vi "RT Driver VI.vi"(7 "Operation":T1, 11 "Device Reference in":T2 format="%.0x") -> (0 "Error Code":i32)   [LabVIEW 2021, in "Software Multi-Plex Engine.lvlib"]
uses:
  Software Multi-Plex Engine.lvlib
  <vilib>/NI VeriStand/Custom Device API/Custom Device Item Ref.ctl
  <vilib>/NI VeriStand/Custom Device API/Hardware Interface Driver VI Operation.ctl
  Shared/Compiled.Settings.ctl
  RTStateVariables.ctl
  <vilib>/NI/NIVS Inline Async API/_VS Inline Async API/VS Inline Async API/VS Inline Async API.lvclass
  <vilib>/NI/NIVS Inline Async API/_VS Inline Async API/VS Inline Async API/VS Inline Async API.lvclass/VS Inline Async API.ctl
  <vilib>/NI/NIVS Inline Async API/_Data Access Engine/Data Access Engine/Data Access Engine.lvclass/Data Access Engine.ctl
  <vilib>/NI/NIVS Inline Async API/_Data Access Engine/Access Type Classes/Write/Write.lvclass/Write.ctl
  <vilib>/NI/NIVS Inline Async API/_Data Access Engine/Access Type Classes/ReadWrite/ReadWrite.lvclass/ReadWrite.ctl
  <vilib>/NI/NIVS Inline Async API/_Data Access Engine/Access Type Classes/Read/Read.lvclass/Read.ctl
  <vilib>/NI/NIVS Inline Async API/_Data Access Engine/Data Access Engine/Methods/Data.Engine.Read Data from HW.vi
  <vilib>/NI/NIVS Inline Async API/_VS Inline Async API/Error Handling Process/SubVIs/Error.GetError.vi
  <vilib>/NI/NIVS Inline Async API/_Data Access Engine/Data Access Engine/Methods/Data.Engine.Write Data to HW.vi
  <vilib>/NI/NIVS Inline Async API/_Data Access Engine/Access Type Classes/ReadWrite/ReadWrite.EngineData.vi
  <vilib>/NI/NIVS Inline Async API/_Data Access Engine/Access Type Classes/Write/Write.EngineData.vi
  <vilib>/NI/NIVS Inline Async API/_Data Access Engine/Access Type Classes/Read/Read.EngineData.vi
  <vilib>/NI VeriStand/Custom Device API/NI VeriStand - Get Channel Value by Data Reference.vi
  <vilib>/NI VeriStand/Custom Device API/NI VeriStand - Set Channel Value by Data Reference.vi
  <vilib>/NI VeriStand/Custom Device API/NI VeriStand - Get Channel Values by Block Data Reference.vi
  Shared/Constants.vi
  <vilib>/NI VeriStand/Custom Device API/Get Item Property (Variant).vi
  <vilib>/NI VeriStand/Custom Device API/Global Data Refs.vi
  <vilib>/NI VeriStand/Custom Device API/Custom Device API.lvlib
  Shared/Software Multi-Plex Shared.lvlib
  <vilib>/NI VeriStand/Custom Device Tools/Custom Device Utility Library/Custom Device Utility Library.lvlib
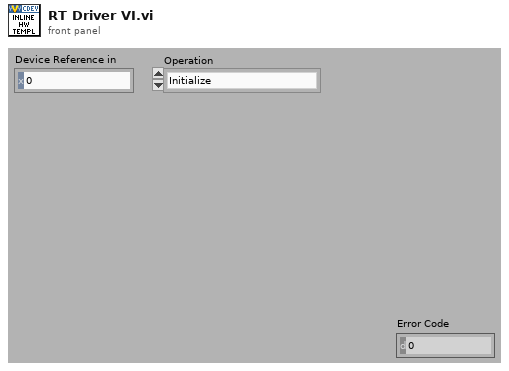
[diagram p1: front panel]
types:
  T1 = typedef "Custom Device API.lvlib/Hardware Interface Driver VI Operation.ctl" = enum16{"Initialize", "Start", "Read Data from HW", "Write Data to HW", "Close"}
  T2 = typedef "Custom Device API.lvlib/Custom Device Item Ref.ctl" = u64
  T3 = typedef "Software Multi-Plex Engine.lvlib/RTStateVariables.ctl" = cluster{"Async":refnum<class "VS Inline Async API.lvclass">, "Settings":T4}
  T4 = typedef "Software Multi-Plex Shared.lvlib/Compiled.Settings.ctl" = cluster{"Name":string, "Number of Channels":i32, "Inputs per Channel":i32, "Global Selector":bool}
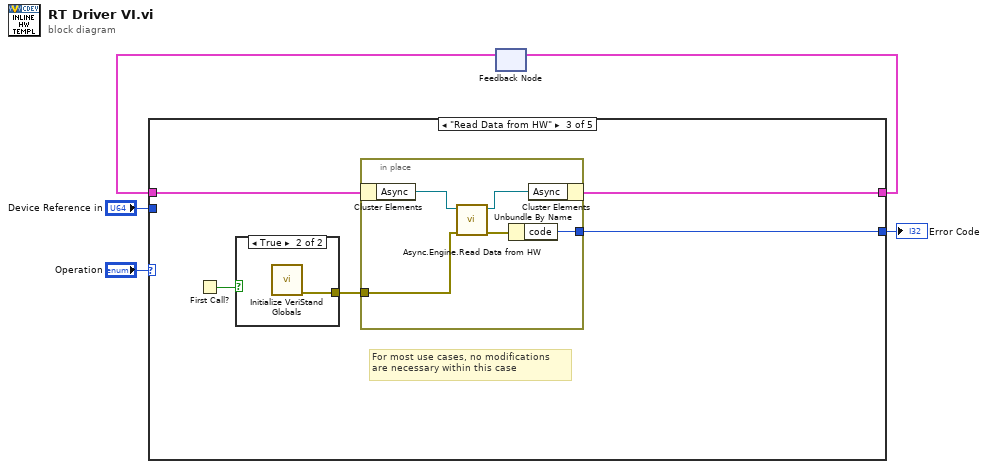
[diagram p0: block diagram]
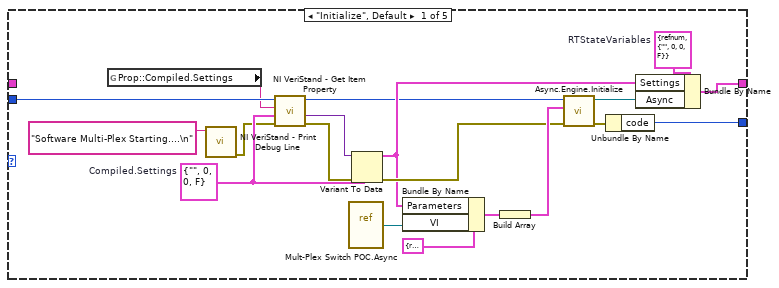
[diagram p2: hidden frame]
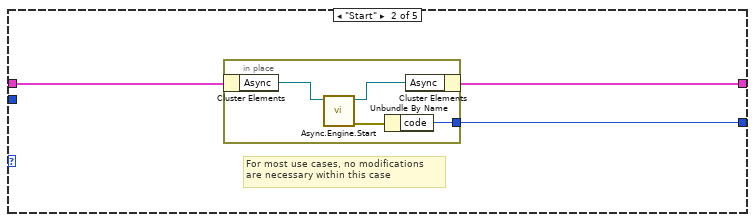
[diagram p3: hidden frame]
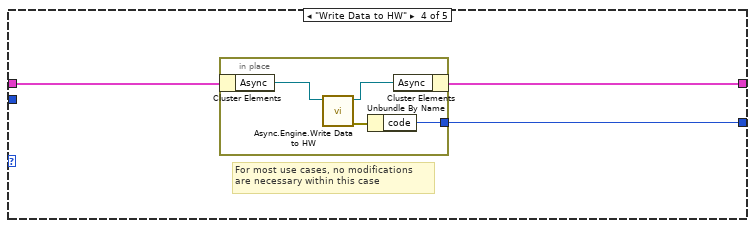
[diagram p5: hidden frame]
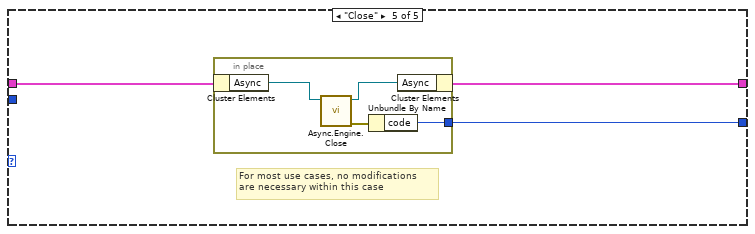
[diagram p6: hidden frame]
diagram:
  n1 = feedback #1() -> (w3:T3)  [unwired: 1 out]
  n2 = case shown="\"Read Data from HW\"" "Operation" {
    tunnel: [w22 w26 w34 w43 w51] -> w4
    tunnel: w3 -> [_ w27 w36 w44 w52]
    tunnel: "Device Reference in" -> [w19 _ _ _ _]
    tunnel: [w24 w25 w35 w45 w50] -> w1
    frame "Initialize", Default {
      w13 = T3 {"Async"=refnum, "Settings"={"Name"="", "Number of Channels"=0, "Inputs per Channel"=0, "Global Selector"=FALSE}}  # RTStateVariables
      w14 = T4 {"Name"="", "Number of Channels"=0, "Inputs per Channel"=0, "Global Selector"=FALSE}  # Compiled.Settings
      n3 = global read "Constants.vi" "Prop::Compiled.Settings"() -> (w16:string)
      n4 = call <vilib>:"NI VeriStand - Print Debug Line.vi"("Message"="Software Multi-Plex Starting....\n") -> ("error out"=w8:errorcluster)  [unwired: 10 in]
      n5 = call-poly <vilib>:"NI VeriStand - Get Item Property.vi"("error in (no error)"=w8, "Default Value"=w14, "Property Name"=w16, "Item Ref in"=w19) -> ("error out"=w18:errorcluster, "Value"=w17:variant, "Item Ref out"=w9:T2)  [unwired: 4 in, 1 out]
      n6 = vi-ref "Mult-Plex Switch POC.Async.vi"() -> (w6:refnum<vi>)
      n7 = Variant To Data(error in=w18, type=w14, Variant=w17) -> (data=w10:T4, error out=w11:errorcluster)
      n8 = Bundle By Name(cluster=cluster{"VI":refnum<vi>, "Parameters":variant} {"VI"=refnum, "Parameters"=variant} ("Process"), "Parameters"=w10, "VI"=w6) -> (w20:cluster{"VI":refnum<vi>, "Parameters":variant})
      n9 = Build Array(w20) -> (w12:cluster{"VI":refnum<vi>, "Parameters":variant}[])
      n10 = call <vilib>:"Async.Engine.Initialize.vi"("error in (no error)"=w11, "Processes"=w12, "Custom Device Ref"=w9) -> ("error out"=w15:errorcluster, "Async"=w23:refnum<class "VS Inline Async API.lvclass">)  [unwired: 7 in]
      n11 = Unbundle By Name(w15) -> ("code"=w24:i32)
      n12 = Bundle By Name(cluster=w13, "Settings"=w10, "Async"=w23) -> (w22:T3)
    }
    frame "Start" {
      # "For most use cases, no modifications \nare necessary within this case"
      n13 = in-place {
        in-place-border: [w28] -> w25
        n14 = in-place-cluster #2(w27) -> ("Async"=w31:refnum<class "VS Inline Async API.lvclass">)
        n15 = call <vilib>:"Async.Engine.Start.vi"("VS Inline Async API in"=w31) -> ("error out"=w29:errorcluster, "VS Inline Async API out"=w30:refnum<class "VS Inline Async API.lvclass">)  [unwired: 9 in]
        n16 = Unbundle By Name(w29) -> ("code"=w28:i32)
        n17 = in-place-cluster #2("Async"=w30) -> (w26:T3)
      }
    }
    frame "Read Data from HW" {
      # "For most use cases, no modifications \nare necessary within this case"
      n18 = First Call?() -> (First Call?: T/F=w33:bool)
      n19 = case shown="True" w33 {
        tunnel: [_ w37] -> w32
        frame False {
        }
        frame True {
          n20 = call "Initialize VeriStand Globals.vi"() -> ("error out"=w37:errorcluster)  [unwired: 11 in]
        }
      }
      n21 = in-place {
        in-place-border: [w40] -> w35
        in-place-border: w32 -> [w38]
        n22 = in-place-cluster #3(w36) -> ("Async"=w42:refnum<class "VS Inline Async API.lvclass">)
        n23 = call <vilib>:"Async.Engine.Read Data from HW.vi"("error in"=w38, "Async in"=w42) -> ("error out"=w39:errorcluster, "Async out"=w41:refnum<class "VS Inline Async API.lvclass">)  [unwired: 8 in]
        n24 = Unbundle By Name(w39) -> ("code"=w40:i32)
        n25 = in-place-cluster #3("Async"=w41) -> (w34:T3)
      }
    }
    frame "Write Data to HW" {
      # "For most use cases, no modifications \nare necessary within this case"
      n26 = in-place {
        in-place-border: [w49] -> w45
        n27 = in-place-cluster #4(w44) -> ("Async"=w47:refnum<class "VS Inline Async API.lvclass">)
        n28 = call <vilib>:"Async.Engine.Write Data to HW.vi"("VS Inline Async API in"=w47) -> ("error out"=w48:errorcluster, "VS Inline Async API out"=w46:refnum<class "VS Inline Async API.lvclass">)  [unwired: 9 in]
        n29 = Unbundle By Name(w48) -> ("code"=w49:i32)
        n30 = in-place-cluster #4("Async"=w46) -> (w43:T3)
      }
    }
    frame "Close" {
      # "For most use cases, no modifications \nare necessary within this case"
      n31 = in-place {
        in-place-border: [w54] -> w50
        n32 = in-place-cluster #5(w52) -> ("Async"=w56:refnum<class "VS Inline Async API.lvclass">)
        n33 = call <vilib>:"Async.Engine.Close.vi"("Async in"=w56) -> ("error out"=w53:errorcluster, "Async out"=w55:refnum<class "VS Inline Async API.lvclass">)  [unwired: 9 in]
        n34 = Unbundle By Name(w53) -> ("code"=w54:i32)
        n35 = in-place-cluster #5("Async"=w55) -> (w51:T3)
      }
    }
  }
  "Error Code" <- w1
  n36 = feedback-in #1(w4) -> ()
